vi "Drivetrain Log Write.vi"(9 "Cluster":T1, 11 "robolog":refnum<k34>) -> ()   [LabVIEW 2013]
uses:
  dashboard/TeleopCmd.ctl
  CmdFlag.ctl
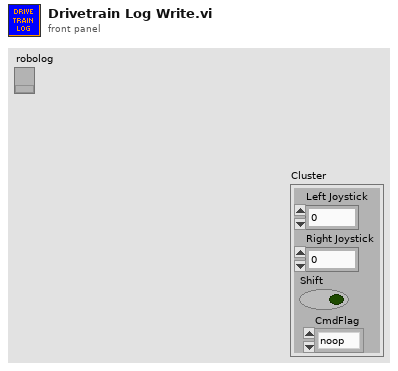
[diagram p1: front panel]
types:
  T1 = typedef "TeleopCmd.ctl" = cluster{"Left Joystick":dbl, "Right Joystick":dbl, "Shift":bool, "CmdFlag":T2}
  T2 = typedef "CmdFlag.ctl" = enum16{"noop", "suspend", "resume"}
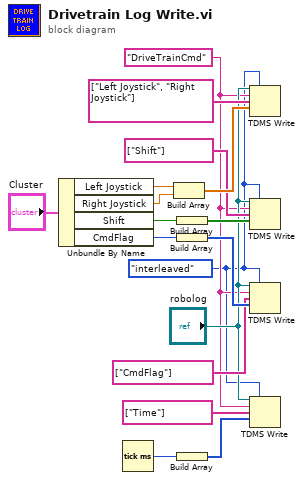
[diagram p0: block diagram]
diagram:
  w1 = enum16{"decimated", "interleaved"}."interleaved" ("data layout (0:decimated)")
  w3 = "DriveTrainCmd" ("group name in (Untitled)")
  n1 = Unbundle By Name("Cluster") -> ("Left Joystick"=w16:dbl, "Right Joystick"=w14:dbl, "Shift"=w12:bool, "CmdFlag"=w7:T2)
  n2 = Tick Count (ms)() -> (millisecond timer value=w5:u32)
  n3 = Build Array(w16, w14) -> (w15:dbl[])
  n4 = Build Array(w12) -> (w11:bool[])
  n5 = Build Array(w7) -> (w9:T2[])
  n6 = Build Array(w5) -> (w4:u32[])
  n7 = TDMS Write(0:"robolog", 1:w1, 5:w3, 7:string[] ["Left Joystick", "Right Joystick"] ("channel name(s) in (Untitled)"), 9:w15) -> ()  [unwired: 1 in, 4 out]
  n8 = TDMS Write(0:"robolog", 1:w1, 5:w3, 7:string[] ["Shift"] ("channel name(s) in (Untitled)"), 9:w11) -> ()  [unwired: 1 in, 4 out]
  n9 = TDMS Write(0:"robolog", 1:w1, 5:w3, 7:string[] ["CmdFlag"] ("channel name(s) in (Untitled)"), 9:w9) -> ()  [unwired: 1 in, 4 out]
  n10 = TDMS Write(0:"robolog", 1:w1, 5:w3, 7:string[] ["Time"] ("channel name(s) in (Untitled)"), 9:w4) -> ()  [unwired: 1 in, 4 out]
